vi "enable disable test 2.vi"() -> ()   [LabVIEW 2019]
panel:
  out "Waveform Chart":dbl(graph)
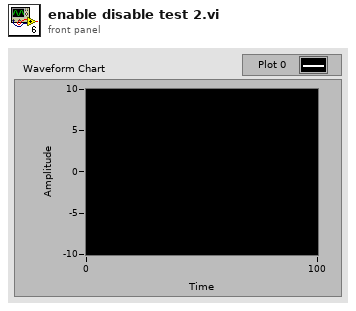
[diagram p1: front panel]
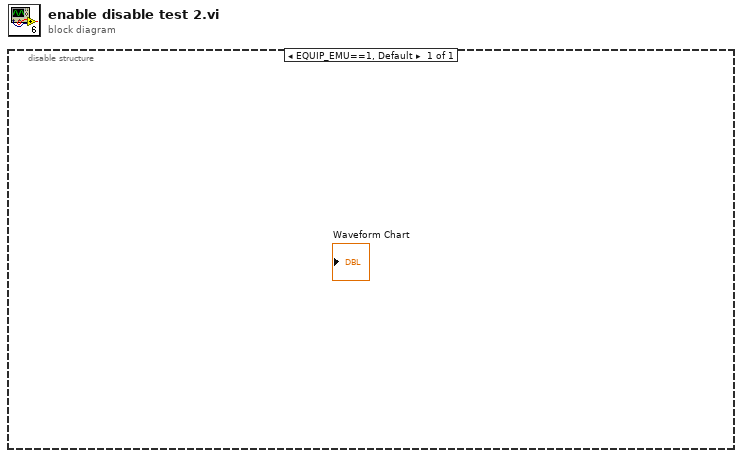
[diagram p0: block diagram]
diagram:
  n1 = disable-structure shown="EQUIP_EMU==1, Default" {
    frame condition #0 (active) {
    }
  }
